vi "Create.vi"(9 "Alias":string, 10 "Actor":refnum<class "Actor.lvclass">, 11 "Dev Actor in":refnum<class "Dev Actor.lvclass">) -> (3 "Dev Actor out":refnum<class "Dev Actor.lvclass">)   [LabVIEW 2021, in "Dev Actor.lvlib" / "Dev Actor.lvclass"]
uses:
  Dev Actor.lvclass
  Actor/Queue Actor/Queue Actor.lvclass
  Actor/Actor/Actor.lvclass
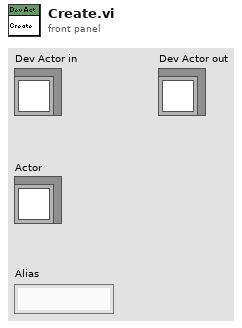
[diagram p1: front panel]
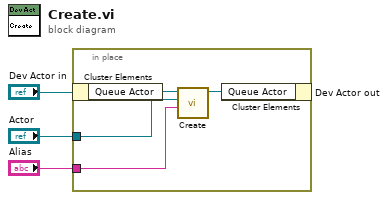
[diagram p0: block diagram]
diagram:
  n1 = in-place {
    in-place-border: "Actor" -> [w5]
    in-place-border: "Alias" -> [w6]
    n2 = in-place-cluster #1("Dev Actor in") -> ("Queue Actor"=w7:refnum<class "Queue Actor.lvclass">)
    n3 = call-dynamic "Create.vi"("Alias"=w6, "Actor"=w5, "Queue Actor in"=w7) -> ("Queue Actor out"=w8:refnum<class "Queue Actor.lvclass">)  [unwired: 8 in]
    n4 = in-place-cluster #1("Queue Actor"=w8) -> (→"Dev Actor out":refnum<class "Dev Actor.lvclass">)
  }
